vi "Group Error IDs.vi"(8 "error in (no error)":errorcluster, 11 "error IDs in":T2[](array[typedef])) -> (0 "error out":errorcluster, 3 "grouped error IDs":T1[](array[typedef]))   [LabVIEW 2017]
uses:
  Error Owner and ID.ctl
  Error Owners and IDs.ctl
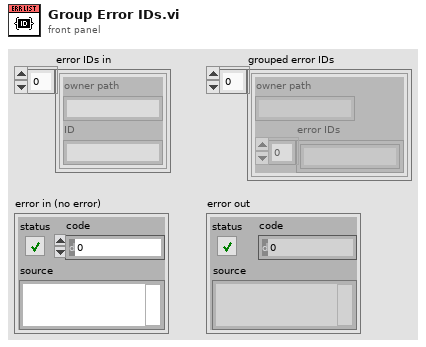
[diagram p1: front panel]
types:
  T1 = typedef "Error Owners and IDs.ctl" = cluster{"owner path":string, "error IDs":string[]}
  T2 = typedef "Error Owner and ID.ctl" = cluster{"owner path":string, "ID":string}
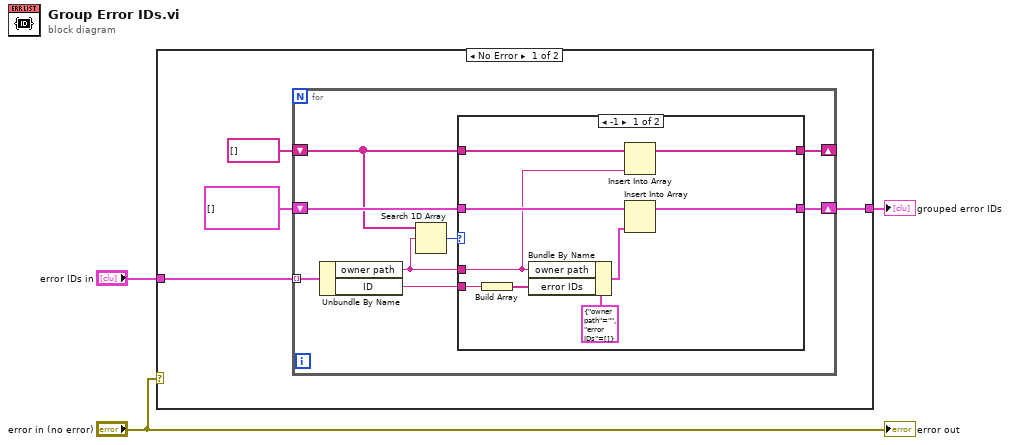
[diagram p0: block diagram]
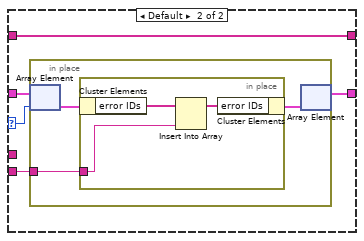
[diagram p2: hidden frame]
diagram:
  n1 = case shown="No Error" "error in (no error)" {
    tunnel: "error IDs in" -> [w7 _]
    tunnel: [w4 _] -> w2
    frame No Error {
      n2 = for {
        tunnel: w7 -> [w15] mode=indexing
        shift-right: [w12] -> w4
        shift-left: T1[] [] ("error IDs") -> [w13]
        shift-right: [w8] -> _
        shift-left: string[] [] -> [w9]
        n3 = Unbundle By Name(w15) -> ("owner path"=w11:string, "ID"=w10:string)
        n4 = Search 1D Array(1D array=w9, element=w11) -> (index of element=w14:i32)  [unwired: 1 in]
        n5 = case shown="-1" w14 {
          selector: w14 -> [_ w28]
          tunnel: w13 -> [w24 w29]
          tunnel: [w23 w27] -> w12
          tunnel: w11 -> [w16 _]
          tunnel: w10 -> [w21 w26]
          tunnel: w9 -> [w18 w25]
          tunnel: [w17 w25] -> w8
          frame -1 {
            n6 = Build Array(w21) -> (w20:string[])
            n7 = Bundle By Name(cluster=T1 {"owner path"="", "error IDs"=[]} ("error"), "owner path"=w16, "error IDs"=w20) -> (w22:T1)
            n8 = Insert Into Array(array=w18, new element=w16) -> (w17:string[])  [unwired: 1 in]
            n9 = Insert Into Array(array=w24, new element=w22) -> (w23:T1[])  [unwired: 1 in]
          }
          frame Default {
            n10 = in-place {
              in-place-border: w26 -> [w30]
              n11 = in-place-array #1(w29, w28) -> (w32:T1)
              n12 = in-place {
                in-place-border: w30 -> [w33]
                n13 = in-place-cluster #2(w32) -> ("error IDs"=w35:string[])
                n14 = Insert Into Array(array=w35, new element=w33) -> (w34:string[])  [unwired: 1 in]
                n15 = in-place-cluster #2("error IDs"=w34) -> (w31:T1)
              }
              n16 = in-place-array #1(w31) -> (w27:T1[])  [unwired: 1 out]
            }
          }
        }
      }
    }
    frame Error {
    }
  }
  "grouped error IDs" <- w2
  "error out" <- "error in (no error)"
